vi "Set Name XML.vi"(1 "Name XML File":string, 2 "Grid in":refnum<class "Grid.lvclass">) -> (0 "Grid out":refnum<class "Grid.lvclass">)   [LabVIEW 2016, in "Grid.lvclass"]
uses:
  Grid.lvclass
  Grid.lvclass/Grid.ctl
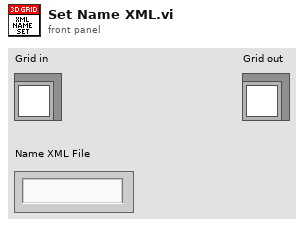
[diagram p1: front panel]
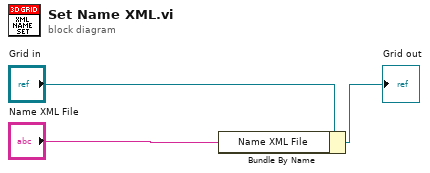
[diagram p0: block diagram]
diagram:
  n1 = Bundle By Name(cluster="Grid in", "Name XML File"="Name XML File") -> (→"Grid out":refnum<class "Grid.lvclass">)
